vi "LVClass_DataServer AddDataID.vi"(0 "DataServer in":refnum<class "DataServer.lvclass">, 5 "name":string, 7 "DataType":T1, 11 "error in (no error)":errorcluster) -> (4 "DataServer out":refnum<class "DataServer.lvclass">, 15 "error out":errorcluster)   [LabVIEW 2020, in "DataServer.lvclass"]
doc: "Set the slopes to be send by TCP connection.\n\n--------------------------------------------------------------------------------\n\n<B>serverIn </B> : Server object.\n<B>serverOut </B> : Server object.\n<B>hasoslopes </B> : HasoSlopes object.\n<B>ErrorIn </B> : Error\n<B>ErrorOut </B> : Error\n\n--------------------------------------------------------------------------------"
uses:
  DataServer.lvclass
  ClientServerDataType.ctl
  ClientServerDataID.ctl
  DataServer.lvclass/DataServer.ctl
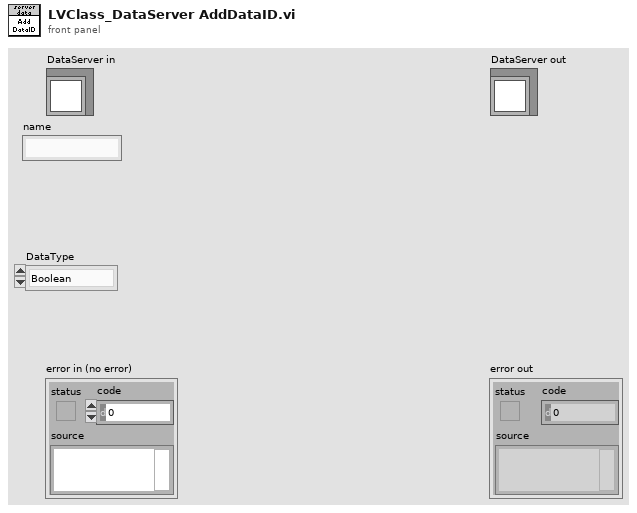
[diagram p1: front panel]
types:
  T1 = typedef "ClientServerDataType.ctl" = enum16{"Boolean", "Integer", "Float", "String", "HasoSlopes", "Image"}
  T2 = typedef "ClientServerDataID.ctl" = cluster{"Name":string, "Type":T1}
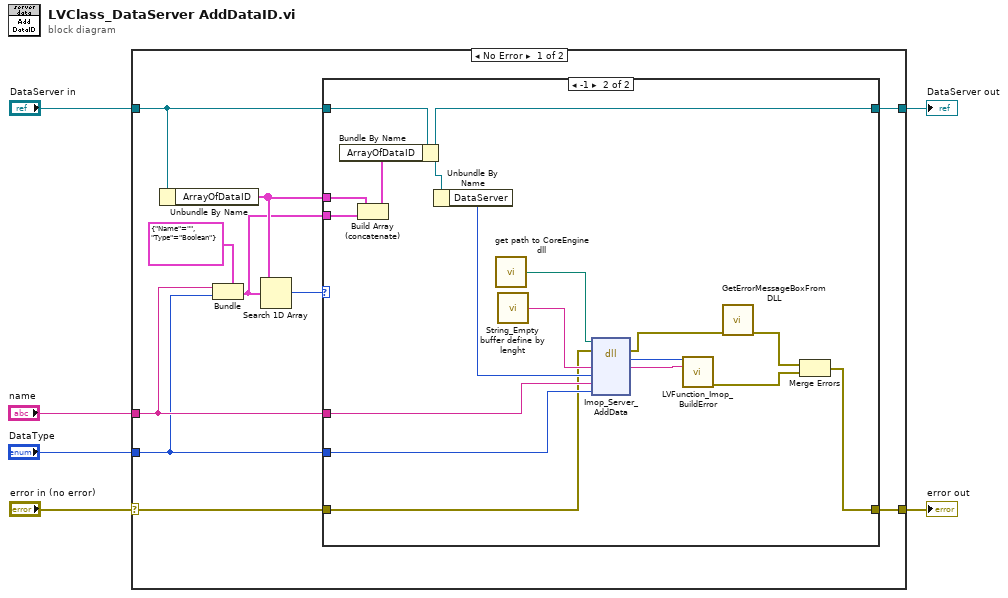
[diagram p0: block diagram]
diagram:
  n1 = case shown="No Error" "error in (no error)" {
    selector: "error in (no error)" -> [w7 w37]
    tunnel: [w16 w37] -> w5
    tunnel: [w12 w36] -> w3
    tunnel: "DataServer in" -> [w11 w36]
    tunnel: "DataType" -> [w14 _]
    tunnel: "name" -> [w15 _]
    frame No Error {
      n2 = Unbundle By Name(w11) -> ("ArrayOfDataID"=w10:T2[])
      n3 = Bundle(cluster=T2 {"Name"="", "Type"=enum."Boolean"} ("DataID"), "Name"=w15, "Type"=w14) -> (w9:T2)
      n4 = Search 1D Array(1D array=w10, element=w9) -> (index of element=w13:i32)  [unwired: 1 in]
      n5 = case shown="-1" w13 {
        tunnel: [w17 w28] -> w16
        tunnel: w15 -> [_ w27]
        tunnel: w14 -> [_ w26]
        tunnel: w11 -> [w18 w25]
        tunnel: [w18 w21] -> w12
        tunnel: w10 -> [_ w24]
        tunnel: w9 -> [_ w23]
        tunnel: w7 -> [w17 w19]
        frame 0, Default {
        }
        frame -1 {
          n6 = Build Array (concatenate)(w24, w23) -> (w22:T2[])
          n7 = Bundle By Name(cluster=w25, "ArrayOfDataID"=w22) -> (w21:refnum<class "DataServer.lvclass">)
          n8 = Unbundle By Name(w21) -> ("DataServer"=w20:i32)
          n9 = call "get path to CoreEngine dll.vi"() -> ("path to c_interface_vc100.dll"=w32:path)  [unwired: 12 in, 3 out]
          n10 = call "String_Empty buffer define by lenght.vi"() -> ("Empty buffer"=w31:string)  [unwired: 1 in]
          n11 = dll-call lib="D:/soft/HASO_v3/SVN_trunk/ImOpCoreEngine4_LV2011/DLLs/c_interface_vc100.dll" fn="Imop_Server_AddData"(path in=w32, error in=w19, "message"=w31, "server"=w20, "name"=w27, "type"=w26) -> (error out=w33:errorcluster, "return type"=w29:i32, "message"=w30:string)  [unwired: 4 in, 1 out]
          n12 = call "LVFunction_Imop_BuildError.vi"("code"=w29, "String to Prepend to source (\"\")"=w30) -> ("error out"=w35:errorcluster)  [unwired: 13 in]
          n13 = call "GetErrorMessageBoxFromDLL.vi"("error IN"=w33) -> ("error OUT"=w34:errorcluster)  [unwired: 10 in]
          n14 = Merge Errors(w34, w35) -> (w28:errorcluster)
        }
      }
    }
    frame Error {
    }
  }
  "error out" <- w5
  "DataServer out" <- w3
